vi "Change Number of Slots and Check.vi"(8 "error in":errorcluster, 9 "number of slots":i32, 10 "chassis ref in":T1 format="%.0x", 11 "test case in":refnum<class "Scan Engine Scripting API Custom Device Unit Tests.lvclass">) -> (0 "error out":errorcluster, 2 "chassis ref out":T1 format="%.0x", 3 "test case out":refnum<class "Scan Engine Scripting API Custom Device Unit Tests.lvclass">)   [LabVIEW 2019]
uses:
  Scripting API/Custom Device/Scan Engine Scripting API Custom Device Unit Tests.lvclass
  <vilib>/NI VeriStand/Custom Device API/Custom Device Item Ref.ctl
  Scripting/Scan Engine Scripting.lvlib
  <vilib>/NI VeriStand/Custom Device API/Custom Device API.lvlib
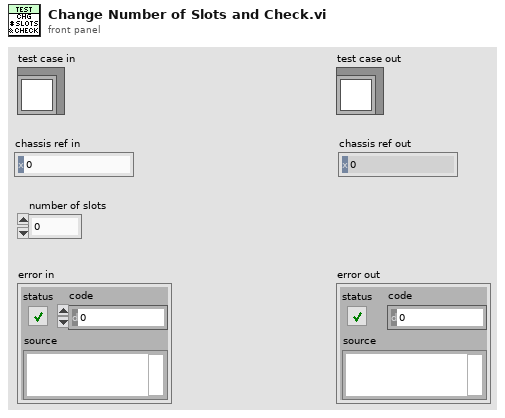
[diagram p1: front panel]
types:
  T1 = typedef "Custom Device API.lvlib/Custom Device Item Ref.ctl" = u64
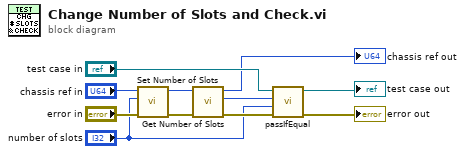
[diagram p0: block diagram]
diagram:
  n1 = call "Set Number of Slots.vi"("error in"="error in", "number of slots"="number of slots", "chassis ref in"="chassis ref in") -> ("error out"=w4:errorcluster, "chassis ref out"=w5:T1)  [unwired: 7 in]
  n2 = call "Get Number of Slots.vi"("error in"=w4, "chassis ref in"=w5) -> ("error out"=w6:errorcluster, "number of slots"=w7:i32, "chassis ref out"=→"chassis ref out":T1)  [unwired: 7 in]
  n3 = call-dynamic "passIfEqual.vi"("error in (no error)"=w6, "y"="number of slots", "x"=w7, "TestCase in"="test case in") -> ("error out"=→"error out":errorcluster, "TestCase out"=→"test case out":refnum<class "Scan Engine Scripting API Custom Device Unit Tests.lvclass">)  [unwired: 6 in]
